vi "Retrieve Actors.vi"(8 "error in (no error)":errorcluster, 11 "Target Store in":refnum<class "Live Store.lvclass">) -> (0 "error out":errorcluster, 1 "Async Methods Actors Paths":path[](array[path]), 2 "Async Methods Actors":string[](array[string]), 3 "Target Store out":refnum<class "Live Store.lvclass">)   [LabVIEW 2023, in "Add Async Methods Actor.lvlib" / "Live Store.lvclass"]
uses:
  Live Store.lvclass
  Live Store.lvclass/Live Store.ctl
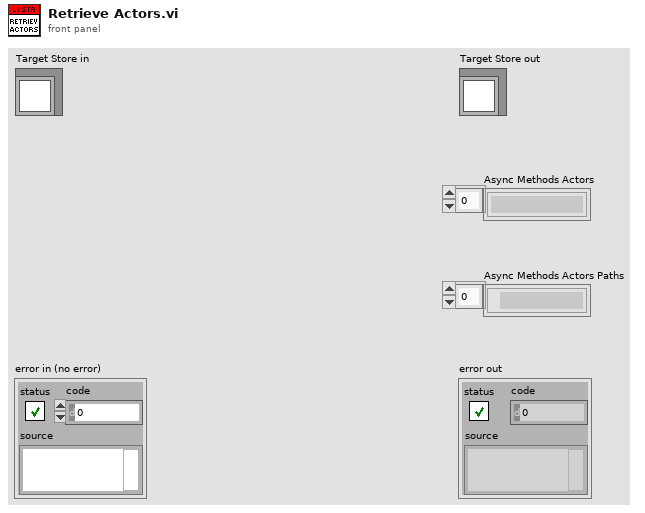
[diagram p1: front panel]
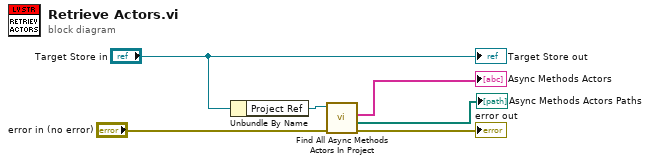
[diagram p0: block diagram]
diagram:
  n1 = Unbundle By Name("Target Store in") -> ("Project Ref"=w3:refnum<vi>)
  n2 = call "Find All Async Methods Actors In Project.vi"("error in (no error)"="error in (no error)", "Project Item in"=w3) -> ("error out"=→"error out":errorcluster, "Async Methods Acotrs Paths"=→"Async Methods Actors Paths":path[], "Async Methods Acotrs Names"=→"Async Methods Actors":string[])  [unwired: 6 in, 1 out]
  "Target Store out" <- "Target Store in"
